vi "RPC_Demo.vi"(11 "Sender":string="RPC Demo") -> ()   [LabVIEW 2014]
uses:
  <vilib>/Utility/miscctls.llb/LVPointTypeDef.ctl
  TSMaster_API/RPC/Typedef/RPC Data.ctl
  <vilib>/Utility/miscctls.llb/LVComboBoxStrsAndValuesArrayTypeDef.ctl
  TSMaster_API/RPC/Typedef/RPC_API_param.ctl
panel:
  out "Connect?":bool
  in  "Disconnect":bool
  in  "TSMaster Proj List":string(combo)
  out "Data out":T1
  in  "选项卡控件":enum32{"Setting", "RPC"}(tab)
  in  "DLL_PATH":path
  in  "API_Call":bool
  in  "API_param":T2
  out "Value":dbl
  in  "Set System Var":bool
  in  "Get System Var":bool
  in  "Var Name":string
  in  "Value_Set":string
  in  "Config":bool
  in  "Connect":bool
  in  "Creat error":bool
  in  "log":i32(listbox)
  in  "Quit":bool
  # "RPC Demo"
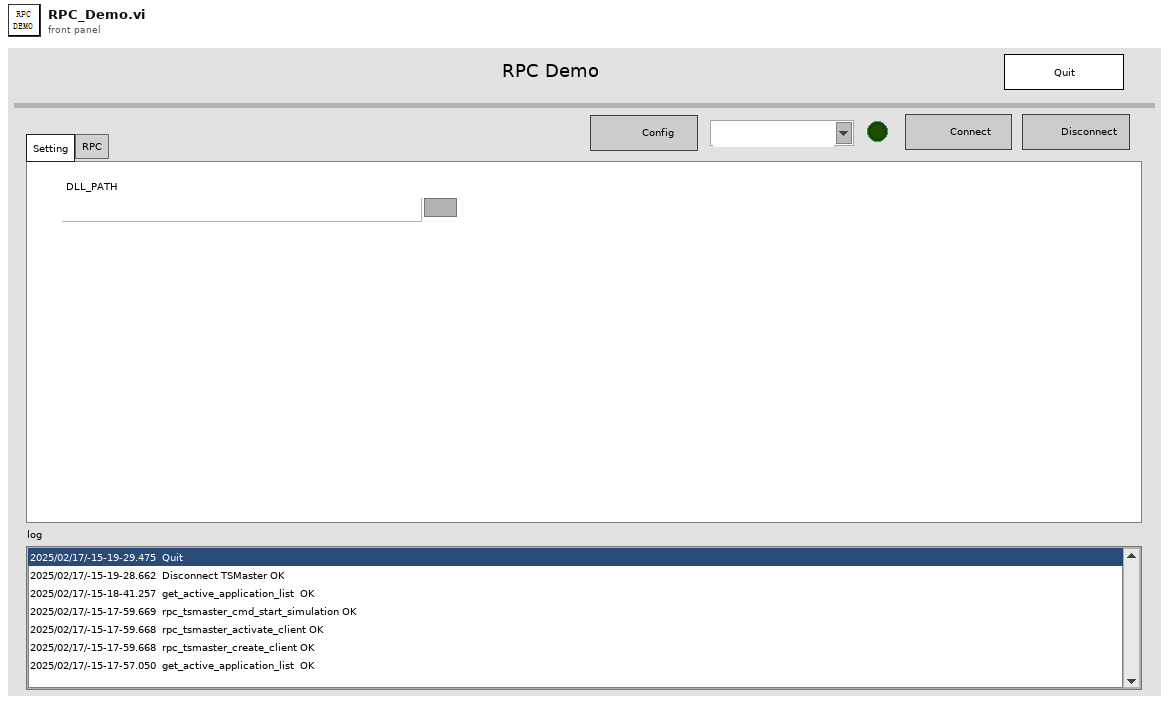
[diagram p1: front panel]
types:
  T1 = typedef "RPC Data.ctl" = cluster{"Communication message":cluster{"Sender":string, "receiver":string, "message":string, "data":variant}, "error in":errorcluster, "Data":cluster{"Config parameter":cluster{"DLL_PATH":path}, "AHandle":i32, "TSMaster Proj":string, "Var Name":string, "API_param":T2}}
  T2 = typedef "RPC_API_param.ctl" = cluster{"AAPIName":string, "AArgCount":i32, "AArgCapacity":i32, "AArgs":string}
  T3 = cluster{"Sender":string, "receiver":string, "message":string, "data":variant}
  T4 = typedef "LVComboBoxStrsAndValuesArrayTypeDef.ctl" = cluster{"String":string, "Value":string}[]
  T5 = typedef "LVPointTypeDef.ctl" = cluster{"Horizontal":i16, "Vertical":i16}
  T6 = cluster{"Config parameter":cluster{"DLL_PATH":path}, "AHandle":i32, "TSMaster Proj":string, "Var Name":string, "API_param":T2}
  T7 = enum32{"invalid app kind", "Development System", "Run Time System", "Student Edition", "Embedded LabVIEW", "Evaluation", "Custom"}
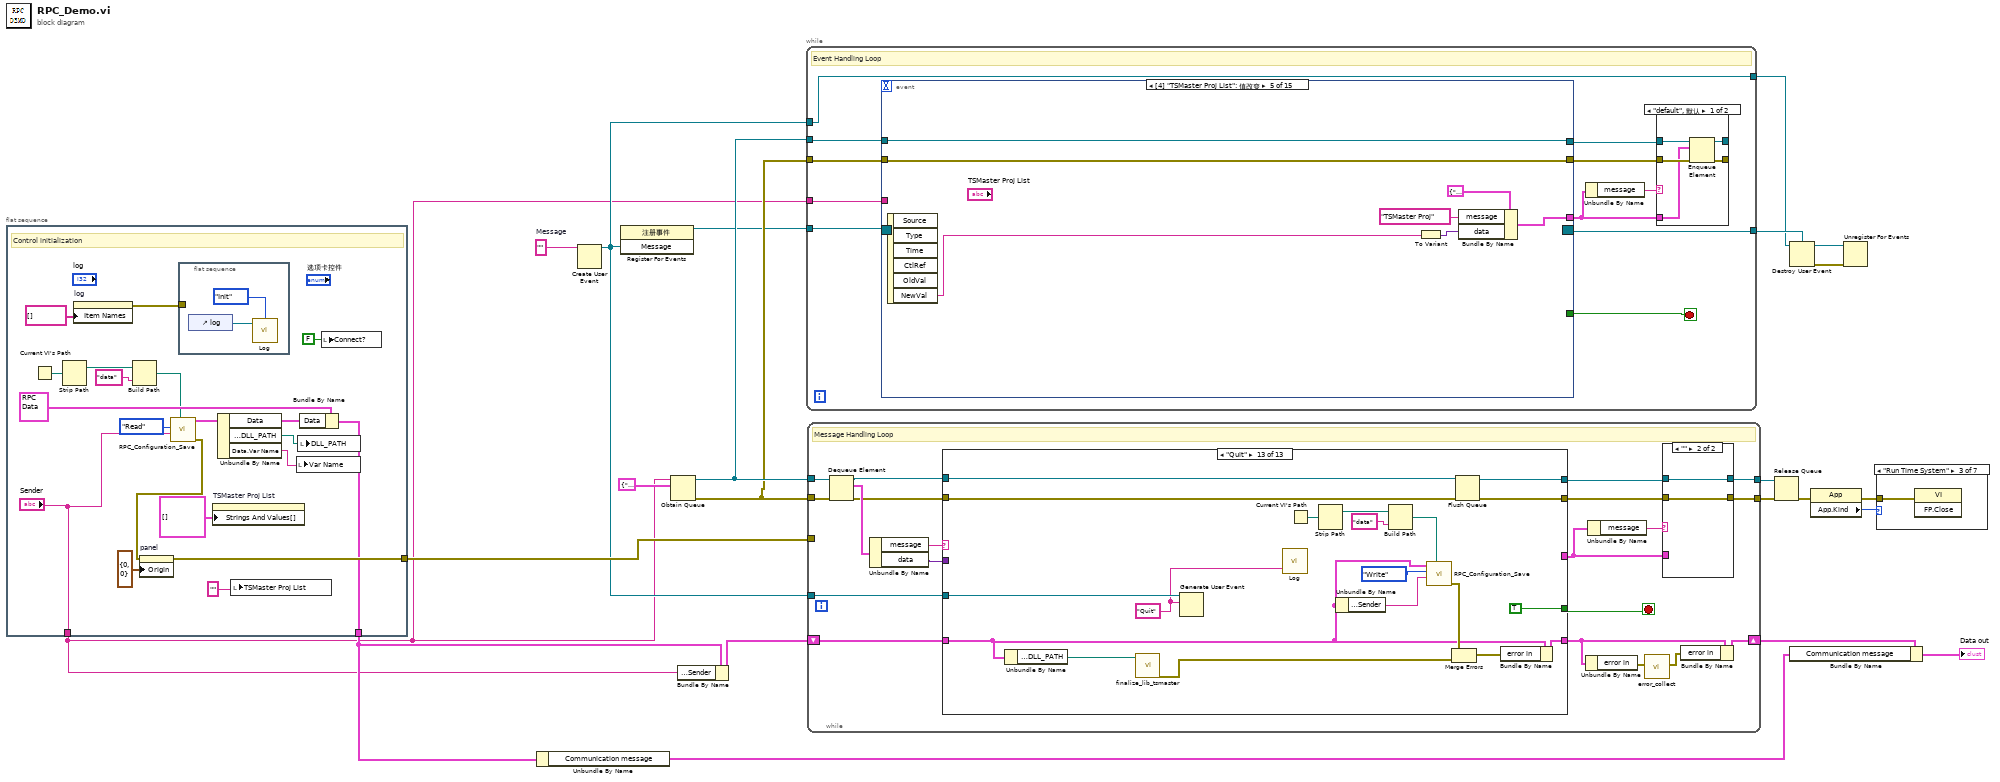
[diagram p0: block diagram]
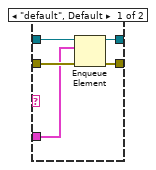
[diagram p8: hidden frame]
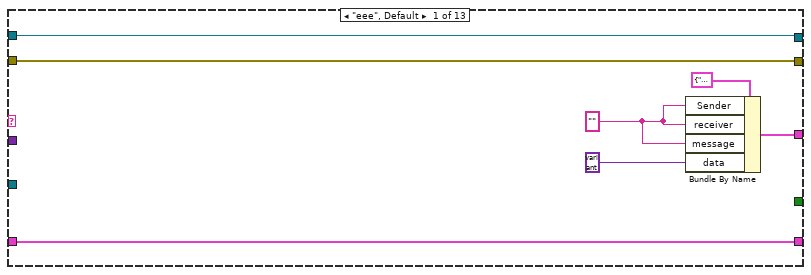
[diagram p9: hidden frame]
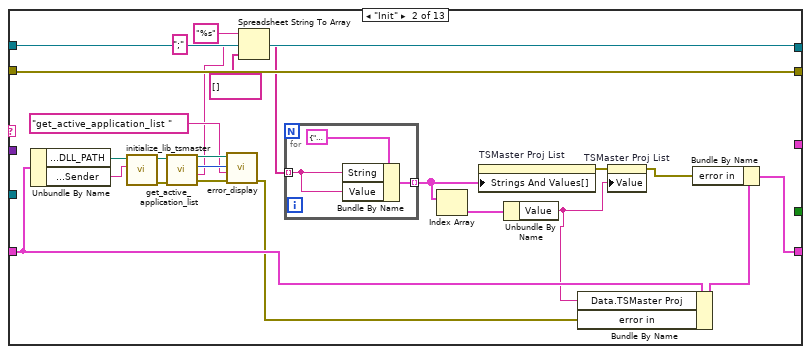
[diagram p10: hidden frame]
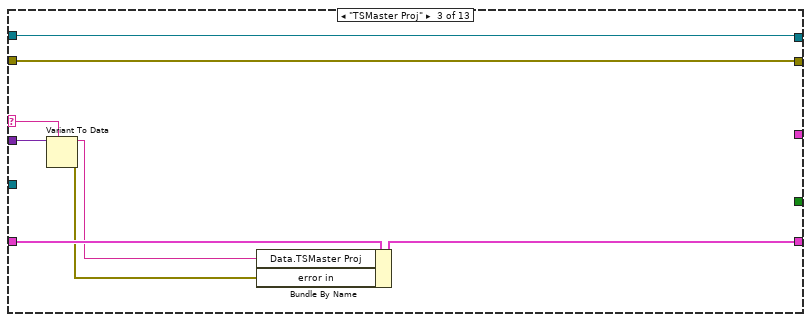
[diagram p11: hidden frame]
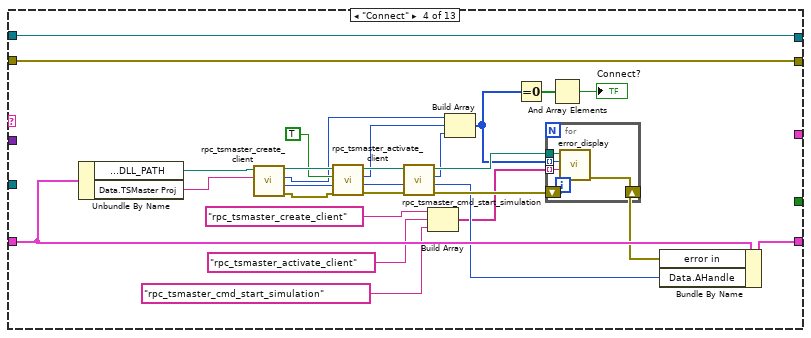
[diagram p12: hidden frame]
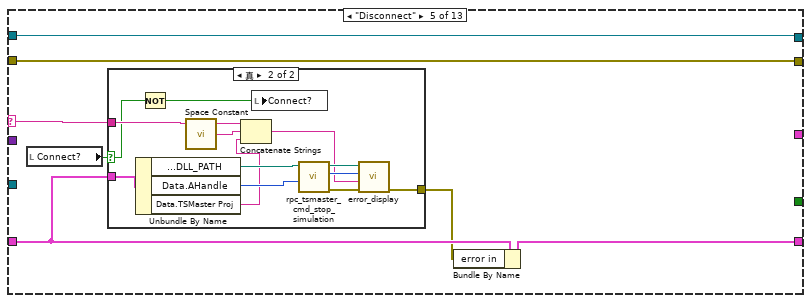
[diagram p13: hidden frame]
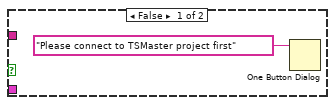
[diagram p14: hidden frame]
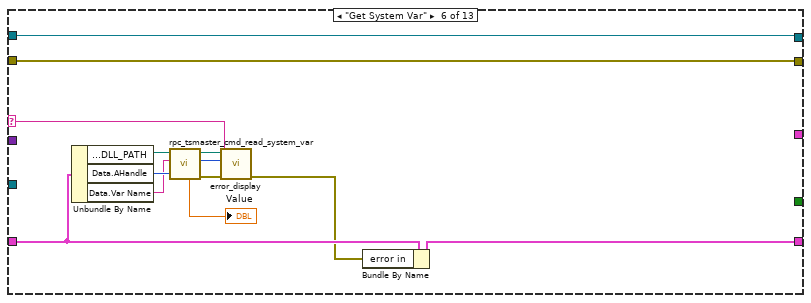
[diagram p15: hidden frame]
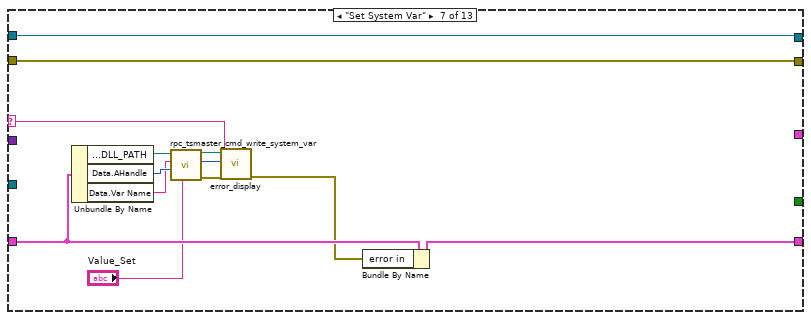
[diagram p16: hidden frame]
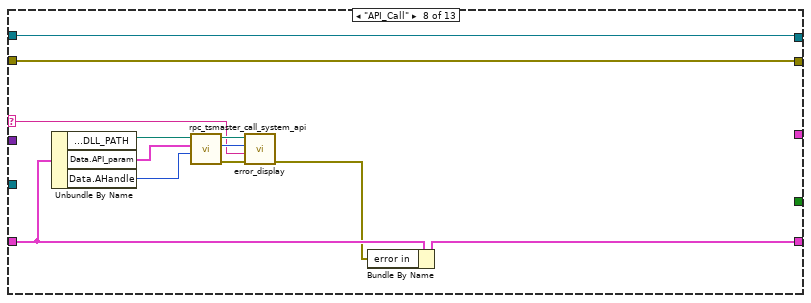
[diagram p17: hidden frame]
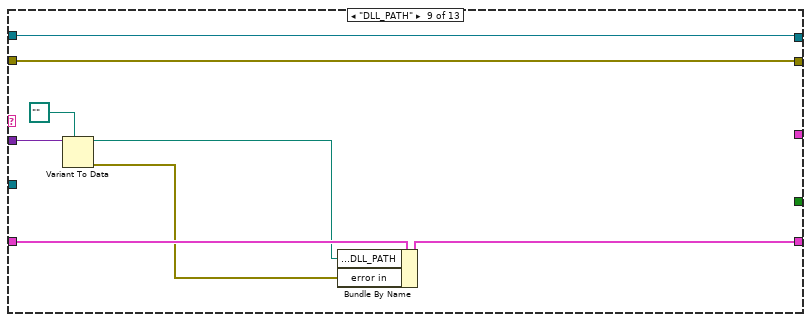
[diagram p18: hidden frame]
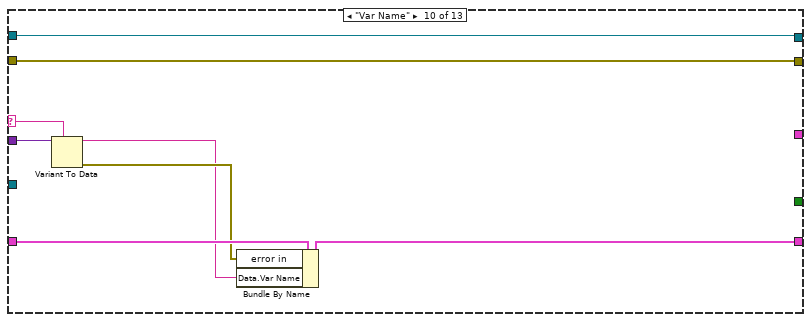
[diagram p19: hidden frame]
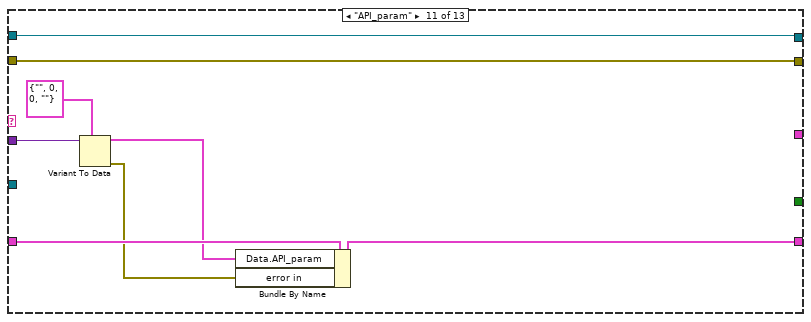
[diagram p20: hidden frame]
diagram:
  w12 = ""  # Message
  n1 = flat-sequence {
    tunnel: [w40] -> w10
    tunnel: [w30] -> w2
    tunnel: ["Sender"] -> w1
    frame #0 {
      # "Control initialization"
      n2 = Current VI's Path() -> (path=w35:path)
      n3 = Strip Path(path=w35) -> (stripped path=w33:path)  [unwired: 1 out]
      n4 = property on="log" class="LstBox (严格)"("Item Names"=string[] [] ("项名")) -> (error out=w38:errorcluster)  [unwired: 2 in, 1 out]
      n5 = Build Path(base path=w33, name or relative path="data") -> (appended path=w32:path)
      n6 = call "RPC_Configuration_Save.vi"("path"=w32, "Config Name"="Sender", "Read/Write"=enum16{"Read", "Write"}."Read") -> ("error in (no error)"=w31:errorcluster, "Data out"=w29:T1)  [unwired: 6 in, 1 out]
      n7 = property on="panel" class="Pane"(error in=w31, "Origin"=T5 {"Horizontal"=0, "Vertical"=0} ("原点")) -> (error out=w40:errorcluster)  [unwired: 1 in, 1 out]
      n8 = flat-sequence {
        tunnel: w38 -> [_]
        frame #0 {
          n9 = control-ref of="log"() -> (w42:refnum<vi>)
          n10 = call "Log.vi"("Method"=enum16{"Init", "Log"}."Init", "ListBox in"=w42) -> ()  [unwired: 2 in]
        }
      }
      n11 = property on="TSMaster Proj List" class="CmbBox"("Strings And Values[]"=T4 [] ("字符串与值[]")) -> ()  [unwired: 2 in, 2 out]
      n12 = Unbundle By Name(w29) -> ("Data"=w28:T6, "Data.Config parameter.DLL_PATH"=w27:path, "Data.Var Name"=w22:string)
      n13 = local write "TSMaster Proj List"("") -> ()
      n14 = local write "Var Name"(w22) -> ()
      n15 = local write "DLL_PATH"(w27) -> ()
      n16 = Bundle By Name(cluster=T1 {"Communication message"={"Sender"="", "receiver"="", "message"="", "data"=variant}, "error in"={"status"=FALSE, "code"=0, "source"=""}, "Data"={"Config parameter"={"DLL_PATH"=path ""}, "AHandle"=0, "TSMaster Proj"="", "Var Name"="", "API_param"={"AAPIName"="", "AArgCount"=0, "AArgCapacity"=0, "AArgs"=""}}} ("Data"), "Data"=w28) -> (w30:T1)
      n17 = local write "Connect?"(FALSE ("Connect?")) -> ()
    }
  }
  n18 = Unbundle By Name(w2) -> ("Communication message"=w4:T3)
  n19 = Create User Event(user event datatype=w12) -> (user event=w7:refnum<user-event>)  [unwired: 1 in, 1 out]
  n20 = register-events(w7) -> (reference out=w11:refnum<event-registration>)  [unwired: 2 in, 1 out]
  n21 = Obtain Queue(name (unnamed)=w1, element data type=T3 {"Sender"="", "receiver"="", "message"="", "data"=variant} ("Communication message")) -> (queue out=w21:refnum<queue>, error out=w14:errorcluster)  [unwired: 3 in, 1 out]
  n22 = Bundle By Name(cluster=w2, "Communication message.Sender"=w1) -> (w13:T1)
  n23 = while {
    tunnel: w21 -> [w53]
    tunnel: w14 -> [w51]
    tunnel: w1 -> [w47]
    tunnel: w11 -> [w46]
    tunnel: [w45] -> w9
    tunnel: w7 -> [w44]
    tunnel: [w44] -> w6
    stop <- w54 stop-if-true
    # "Event Handling Loop"
    n24 = event shown="[4] \"TSMaster Proj List\": 值改变" {
      selector: w46 -> [_ _ _ _ _ _ _ _ _ _ _ _ _ _ _]
      dyn-events: [_ _ _ _ _ _ _ _ _ _ _ _ _ _ _] -> w45
      timeout: _ -> [_ _ _ _ _ _ _ _ _ _ _ _ _ _ _]
      tunnel: [_ _ _ _ _ _ _ _ _ _ _ _ w129 w134 _] -> w54
      tunnel: w53 -> [w64 w71 w78 w83 w90 w95 w100 w105 w110 w115 w122 w127 w132 w137 w144]
      tunnel: [w64 w71 w78 w83 w90 w95 w100 w105 w110 w115 w122 w127 w132 w135 w144] -> w52
      tunnel: [T3 {"Sender"="", "receiver"="", "message"="", "data"=variant} ("Communication message") w67 w73 w79 w86 w91 w96 w101 w106 w111 w118 w125 _ _ w140] -> w49
      tunnel: [w63 w70 w77 w82 w89 w94 w99 w104 w109 w114 w121 w123 w128 w133 w143] -> w50
      tunnel: w51 -> [w63 w70 w77 w82 w89 w94 w99 w104 w109 w114 w121 w123 w128 w133 w143]
      tunnel: w47 -> [_ _ _ _ _ _ _ _ _ _ _ _ _ _ _]
      event Timeout {
        n25 = event-data() -> ()  [unwired: 1 in, 3 out]
      }
      event "DLL_PATH": Value Change {
        n26 = event-data() -> ("NewVal"=w65:path)  [unwired: 1 in, 5 out]
        n27 = To Variant(anything=w65) -> (Variant=w66:variant)
        n28 = Bundle By Name(cluster=T3 {"Sender"="", "receiver"="", "message"="", "data"=variant} ("Communication message"), "message"="DLL_PATH" ("Sender"), "data"=w66) -> (w67:T3)
      }
      event "Var Name": Value Change {
        n29 = event-data() -> ("NewVal"=w72:string)  [unwired: 1 in, 5 out]
        n30 = To Variant(anything=w72) -> (Variant=w74:variant)
        n31 = Bundle By Name(cluster=T3 {"Sender"="", "receiver"="", "message"="", "data"=variant} ("Communication message"), "message"="Var Name" ("Sender"), "data"=w74) -> (w73:T3)
      }
      event "Config": Value Change {
        n32 = event-data() -> ()  [unwired: 1 in, 6 out]
        n33 = Bundle By Name(cluster=T3 {"Sender"="", "receiver"="", "message"="", "data"=variant} ("Communication message"), "message"="Init" ("Sender")) -> (w79:T3)
      }
      event "TSMaster Proj List": Value Change {
        n34 = event-data() -> ("NewVal"=w84:string)  [unwired: 1 in, 5 out]
        n35 = To Variant(anything=w84) -> (Variant=w85:variant)
        n36 = Bundle By Name(cluster=T3 {"Sender"="", "receiver"="", "message"="", "data"=variant} ("Communication message"), "message"="TSMaster Proj" ("Sender"), "data"=w85) -> (w86:T3)
      }
      event "Connect": Value Change {
        n37 = event-data() -> ()  [unwired: 1 in, 6 out]
        n38 = Bundle By Name(cluster=T3 {"Sender"="", "receiver"="", "message"="", "data"=variant} ("Communication message"), "message"="Connect" ("Sender")) -> (w91:T3)
      }
      event "Disconnect": Value Change {
        n39 = event-data() -> ()  [unwired: 1 in, 6 out]
        n40 = Bundle By Name(cluster=T3 {"Sender"="", "receiver"="", "message"="", "data"=variant} ("Communication message"), "message"="Disconnect" ("Sender")) -> (w96:T3)
      }
      event "Get System Var": Value Change {
        n41 = event-data() -> ()  [unwired: 1 in, 1 out]
        n42 = Bundle By Name(cluster=T3 {"Sender"="", "receiver"="", "message"="", "data"=variant} ("Communication message"), "message"="Get System Var" ("Sender")) -> (w101:T3)
      }
      event "Set System Var": Value Change {
        n43 = event-data() -> ()  [unwired: 1 in, 6 out]
        n44 = Bundle By Name(cluster=T3 {"Sender"="", "receiver"="", "message"="", "data"=variant} ("Communication message"), "message"="Set System Var" ("Sender")) -> (w106:T3)
      }
      event "API_Call": Value Change {
        n45 = event-data() -> ()  [unwired: 1 in, 6 out]
        n46 = Bundle By Name(cluster=T3 {"Sender"="", "receiver"="", "message"="", "data"=variant} ("Communication message"), "message"="API_Call" ("Sender")) -> (w111:T3)
      }
      event Value Change {
        n47 = event-data() -> ("NewVal"=w116:T2)  [unwired: 1 in, 5 out]
        n48 = To Variant(anything=w116) -> (Variant=w117:variant)
        n49 = Bundle By Name(cluster=T3 {"Sender"="", "receiver"="", "message"="", "data"=variant} ("Communication message"), "message"="API_param" ("Sender"), "data"=w117) -> (w118:T3)
      }
      event "Quit": Value Change {
        n50 = event-data() -> ()  [unwired: 1 in, 6 out]
        n51 = Bundle By Name(cluster=T3 {"Sender"="", "receiver"="", "message"="", "data"=variant} ("Communication message"), "message"="Quit" ("Sender")) -> (w125:T3)
      }
      event User Event {
        n52 = event-data() -> ("Message"=w131:string)  [unwired: 1 in]
        n53 = Equal?(x=w131, y="Quit") -> (x = y?=w129:bool)
      }
      event Panel Close? {
        w134 = TRUE ("放弃？")
        n54 = event-data() -> ()  [unwired: 1 in, 4 out]
        n55 = Enqueue Element(queue=w137, element=T3 {"Sender"="", "receiver"="", "message"="Quit", "data"=variant} ("Communication message")) -> (queue out=w135:refnum<queue>)  [unwired: 2 in, 2 out]
        n56 = event-data("Discard?"=w134) -> ()  [unwired: 1 in, 1 out]
      }
      event "Creat error": Value Change {
        n57 = event-data() -> ()  [unwired: 1 in, 6 out]
        n58 = To Variant(anything=errorcluster {"status"=TRUE, "code"=709394, "source"="This is a error demo"}) -> (Variant=w138:variant)
        n59 = Bundle By Name(cluster=T3 {"Sender"="", "receiver"="", "message"="", "data"=variant} ("Communication message"), "message"="Creat error" ("Sender"), "data"=w138) -> (w140:T3)
      }
    }
    n60 = Unbundle By Name(w49) -> ("message"=w48:string)
    n61 = case shown="\"default\", 默认" w48 {
      tunnel: w52 -> [w59 w61]
      tunnel: w50 -> [w58 w60]
      tunnel: w49 -> [w57 _]
      tunnel: [w56 w61] -> _
      tunnel: [w55 w60] -> _
      frame "default", Default {
        n62 = Enqueue Element(queue=w59, element=w57, error in (no error)=w58) -> (queue out=w56:refnum<queue>, error out=w55:errorcluster)  [unwired: 1 in, 1 out]
      }
      frame "" {
      }
    }
  }
  n63 = while {
    tunnel: w21 -> [w164]
    tunnel: w14 -> [w163]
    tunnel: [w155] -> w20
    tunnel: [w154] -> w19
    shift-right: [w146] -> w5
    shift-left: w13 -> [w150]
    tunnel: w10 -> [_]
    tunnel: w7 -> [w149]
    stop <- w153 stop-if-true
    # "Message Handling Loop"
    n64 = Dequeue Element(queue=w164, error in (no error)=w163) -> (queue out=w160:refnum<queue>, element=w162:T3, error out=w159:errorcluster)  [unwired: 1 in, 1 out]
    n65 = Unbundle By Name(w162) -> ("message"=w161:string, "data"=w156:variant)
    n66 = case shown="\"Quit\"" w161 {
      selector: w161 -> [_ _ w209 _ w249 w271 w289 w295 _ w316 _ _ _]
      tunnel: [w178 w202 w213 w240 w252 w279 w292 w304 w312 w320 w328 w335 w353] -> w158
      tunnel: w160 -> [w178 w202 w213 w240 w252 w279 w292 w304 w312 w320 w328 w335 w352]
      tunnel: w159 -> [w177 w201 w212 w239 w251 w278 w291 w303 w311 w319 w327 w334 w350]
      tunnel: [w177 w201 w212 w239 w251 w278 w291 w303 w311 w319 w327 w334 w351] -> w157
      tunnel: w156 -> [_ _ w210 _ _ _ _ _ w309 w317 w325 w332 _]
      tunnel: [_ _ _ _ _ _ _ _ _ _ _ _ TRUE] -> w153
      tunnel: [w175 _ _ _ _ _ _ _ _ _ _ _ _] -> w152
      tunnel: [w172 w192 w208 w227 w248 w270 w288 w294 w307 w315 w323 w330 w342] -> w148
      tunnel: w150 -> [w172 w200 w211 w238 w250 w277 w290 w302 w310 w318 w326 w333 w339]
      tunnel: w149 -> [_ _ _ _ _ _ _ _ _ _ _ _ w349]
      frame "eee", Default {
        w173 = ""
        n67 = Bundle By Name(cluster=T3 {"Sender"="", "receiver"="", "message"="", "data"=variant} ("Communication message"), "Sender"=w173, "receiver"=w173, "message"=w173, "data"=variant) -> (w175:T3)
      }
      frame "Init" {
        n68 = Unbundle By Name(w200) -> ("Data.Config parameter.DLL_PATH"=w199:path, "Communication message.Sender"=w198:string)
        n69 = call "initialize_lib_tsmaster.vi"("AppName"=w198, "Path input"=w199) -> ("error output"=w196:errorcluster, "Path output"=w197:path)  [unwired: 8 in]
        n70 = call "get_active_application_list.vi"("error in"=w196, "path in"=w197) -> ("error out"=w194:errorcluster, "ATSMasterAppNames"=w187:string, "return"=w193:i32, "path out"=w195:path)  [unwired: 6 in]
        n71 = call "error_display.vi"("error in"=w194, "Action name"="get_active_application_list ", "return"=w193, "DLL path"=w195) -> ("error out"=w179:errorcluster)  [unwired: 6 in, 1 out]
        n72 = Spreadsheet String To Array(delimiter (Tab)=";" ("分隔符(Tab)"), format string="%s", spreadsheet string=w187, array type (2D Dbl)=string[] []) -> (array=w186:string[])
        n73 = for {
          tunnel: w186 -> [w204] mode=indexing
          tunnel: [w203] -> w184 mode=indexing
          n74 = Bundle By Name(cluster=cluster{"String":string, "Value":string} {"String"="", "Value"=""}, "String"=w204, "Value"=w204) -> (w203:cluster{"String":string, "Value":string})
        }
        n75 = Index Array(array=w184) -> (element=w183:cluster{"String":string, "Value":string})  [unwired: 1 in]
        n76 = property on="TSMaster Proj List" class="CmbBox"("Strings And Values[]"=w184) -> (error out=w185:errorcluster)  [unwired: 2 in, 1 out]
        n77 = Unbundle By Name(w183) -> ("Value"=w180:string)
        n78 = Bundle By Name(cluster=w200, "Data.TSMaster Proj"=w180, "error in"=w179) -> (w181:T1)
        n79 = property on="TSMaster Proj List" class="CmbBox"(error in=w185, "Value"=w180) -> (error out=w182:errorcluster)  [unwired: 1 in, 1 out]
        n80 = Bundle By Name(cluster=w181, "error in"=w182) -> (w192:T1)
      }
      frame "TSMaster Proj" {
        n81 = Variant To Data(type=w209, Variant=w210) -> (data=w207:string, error out=w206:errorcluster)  [unwired: 1 in]
        n82 = Bundle By Name(cluster=w211, "Data.TSMaster Proj"=w207, "error in"=w206) -> (w208:T1)
      }
      frame "Connect" {
        n83 = Unbundle By Name(w238) -> ("Data.Config parameter.DLL_PATH"=w237:path, "Data.TSMaster Proj"=w217:string)
        n84 = call "rpc_tsmaster_create_client.vi"("AppName"=w217, "Path input"=w237) -> ("error output"=w234:errorcluster, "AHandle"=w231:i32, "return"=w224:i32, "Path output"=w236:path)  [unwired: 6 in]
        n85 = call "rpc_tsmaster_activate_client.vi"("error in (no error)"=w234, "AHandle"=w231, "AActivate"=TRUE, "Path input"=w236) -> ("error output"=w233:errorcluster, "AHandle 2"=w229:i32, "return"=w223:i32, "Path output"=w235:path)  [unwired: 4 in]
        n86 = call "rpc_tsmaster_cmd_start_simulation.vi"("error in (no error)"=w233, "AHandle"=w229, "路径输入"=w235) -> ("error out"=w232:errorcluster, "AHandle 2"=w225:u32, "return"=w222:i32, "路径输出"=w228:path)  [unwired: 5 in]
        n87 = Build Array("rpc_tsmaster_create_client", "rpc_tsmaster_activate_client", "rpc_tsmaster_cmd_start_simulation") -> (w218:string[])
        n88 = Build Array(w224, w223, w222) -> (w216:i32[])
        n89 = Equal To 0?(x=w216) -> (x = 0?=w215:bool[])
        n90 = for {
          tunnel: w228 -> [w244]
          shift-right: [w243] -> w226
          shift-left: w232 -> [w245]
          tunnel: w216 -> [w242] mode=indexing
          tunnel: w218 -> [w241] mode=indexing
          n91 = call "error_display.vi"("error in"=w245, "Action name"=w241, "return"=w242, "DLL path"=w244) -> ("error out"=w243:errorcluster)  [unwired: 6 in, 1 out]
        }
        n92 = And Array Elements(Boolean array=w215) -> (logical AND=→"Connect?":bool)
        n93 = Bundle By Name(cluster=w238, "error in"=w226, "Data.AHandle"=w225) -> (w227:T1)
      }
      frame "Disconnect" {
        n94 = local read "Connect?"() -> (w246:bool)
        n95 = case shown="真" w246 {
          selector: w246 -> [_ w255]
          tunnel: w250 -> [_ w266]
          tunnel: w249 -> [_ w260]
          tunnel: [_ w259] -> w247
          frame False {
            n96 = One Button Dialog(message="Please connect to TSMaster project first" ("消息")) -> ()  [unwired: 1 in, 1 out]
          }
          frame True {
            n97 = Unbundle By Name(w266) -> ("Data.Config parameter.DLL_PATH"=w265:path, "Data.AHandle"=w264:i32, "Data.TSMaster Proj"=w257:string)
            n98 = Not(x=w255) -> (.not. x?=w254:bool)
            n99 = call <vilib>:"Space Constant.vi"() -> ("String"=w256:string)
            n100 = Concatenate Strings(w260, w256, w257) -> (w258:string)
            n101 = local write "Connect?"(w254) -> ()
            n102 = call "rpc_tsmaster_cmd_stop_simulation.vi"("AHandle"=w264, "路径输入"=w265) -> ("error out"=w262:errorcluster, "function return"=w261:i32, "路径输出"=w263:path)  [unwired: 7 in]
            n103 = call "error_display.vi"("error in"=w262, "Action name"=w258, "return"=w261, "DLL path"=w263) -> ("error out"=w259:errorcluster)  [unwired: 6 in, 1 out]
          }
        }
        n104 = Bundle By Name(cluster=w250, "error in"=w247) -> (w248:T1)
      }
      frame "Get System Var" {
        n105 = Unbundle By Name(w277) -> ("Data.Config parameter.DLL_PATH"=w276:path, "Data.AHandle"=w275:i32, "Data.Var Name"=w267:string)
        n106 = call "rpc_tsmaster_cmd_read_system_var.vi"("AHandle"=w275, "ASysVarName"=w267, "Path input"=w276) -> ("error output"=w274:errorcluster, "return"=w272:i32, "Path output"=w273:path, "AValue"=→"Value":dbl)  [unwired: 4 in, 1 out]
        n107 = call "error_display.vi"("error in"=w274, "Action name"=w271, "return"=w272, "DLL path"=w273) -> ("error out"=w269:errorcluster)  [unwired: 6 in, 1 out]
        n108 = Bundle By Name(cluster=w277, "error in"=w269) -> (w270:T1)
      }
      frame "Set System Var" {
        n109 = Unbundle By Name(w290) -> ("Data.Config parameter.DLL_PATH"=w286:path, "Data.AHandle"=w281:i32, "Data.Var Name"=w280:string)
        n110 = call "rpc_tsmaster_cmd_write_system_var.vi"("AValue"="Value_Set", "AHandle"=w281, "ACompleteName"=w280, "Path input"=w286) -> ("error output"=w284:errorcluster, "return"=w283:i32, "Path output"=w285:path)  [unwired: 4 in, 1 out]
        n111 = call "error_display.vi"("error in"=w284, "Action name"=w289, "return"=w283, "DLL path"=w285) -> ("error out"=w287:errorcluster)  [unwired: 6 in, 1 out]
        n112 = Bundle By Name(cluster=w290, "error in"=w287) -> (w288:T1)
      }
      frame "API_Call" {
        n113 = Unbundle By Name(w302) -> ("Data.Config parameter.DLL_PATH"=w301:path, "Data.API_param"=w300:T2, "Data.AHandle"=w299:i32)
        n114 = call "rpc_tsmaster_call_system_api.vi"("AHandle"=w299, "API_param"=w300, "路径输入"=w301) -> ("error out"=w296:errorcluster, "function return"=w297:i32, "路径输出"=w298:path)  [unwired: 6 in]
        n115 = call "error_display.vi"("error in"=w296, "Action name"=w295, "return"=w297, "DLL path"=w298) -> ("error out"=w293:errorcluster)  [unwired: 6 in, 1 out]
        n116 = Bundle By Name(cluster=w302, "error in"=w293) -> (w294:T1)
      }
      frame "DLL_PATH" {
        n117 = Variant To Data(type=path "" ("DLL_PATH"), Variant=w309) -> (data=w306:path, error out=w305:errorcluster)  [unwired: 1 in]
        n118 = Bundle By Name(cluster=w310, "Data.Config parameter.DLL_PATH"=w306, "error in"=w305) -> (w307:T1)
      }
      frame "Var Name" {
        n119 = Variant To Data(type=w316, Variant=w317) -> (data=w313:string, error out=w314:errorcluster)  [unwired: 1 in]
        n120 = Bundle By Name(cluster=w318, "error in"=w314, "Data.Var Name"=w313) -> (w315:T1)
      }
      frame "API_param" {
        n121 = Variant To Data(type=T2 {"AAPIName"="", "AArgCount"=0, "AArgCapacity"=0, "AArgs"=""} ("API_param"), Variant=w325) -> (data=w322:T2, error out=w321:errorcluster)  [unwired: 1 in]
        n122 = Bundle By Name(cluster=w326, "Data.API_param"=w322, "error in"=w321) -> (w323:T1)
      }
      frame "Creat error" {
        n123 = Variant To Data(type=errorcluster {"status"=FALSE, "code"=0, "source"=""} ("error out"), Variant=w332) -> (data=w329:errorcluster)  [unwired: 1 in, 1 out]
        n124 = Bundle By Name(cluster=w333, "error in"=w329) -> (w330:T1)
      }
      frame "Quit" {
        w348 = "Quit" ("y")
        n125 = Unbundle By Name(w339) -> ("Data.Config parameter.DLL_PATH"=w338:path)
        n126 = call "finalize_lib_tsmaster.vi"("Path"=w338) -> ("error out"=w336:errorcluster)  [unwired: 9 in, 1 out]
        n127 = Generate User Event(user event=w349, event data cluster=w348) -> ()  [unwired: 2 in, 2 out]
        n128 = call "Log.vi"("Data"=w348) -> ()  [unwired: 3 in]
        n129 = Current VI's Path() -> (path=w344:path)
        n130 = Strip Path(path=w344) -> (stripped path=w346:path)  [unwired: 1 out]
        n131 = Unbundle By Name(w339) -> ("Communication message.Sender"=w340:string)
        n132 = Build Path(base path=w346, name or relative path="data") -> (appended path=w347:path)
        n133 = call "RPC_Configuration_Save.vi"("path"=w347, "Config Name"=w340, "Read/Write"=enum16{"Read", "Write"}."Write", "Data in"=w339) -> ("error in (no error)"=w341:errorcluster)  [unwired: 5 in, 2 out]
        n134 = Merge Errors(w341, w336) -> (w337:errorcluster)
        n135 = Flush Queue(queue=w352, error in (no error)=w350) -> (queue out=w353:refnum<queue>, error out=w351:errorcluster)  [unwired: 1 out]
        n136 = Bundle By Name(cluster=w339, "error in"=w337) -> (w342:T1)
      }
    }
    n137 = Unbundle By Name(w148) -> ("error in"=w147:errorcluster)
    n138 = Unbundle By Name(w152) -> ("message"=w151:string)
    n139 = call "error_collect.vi"("error in (no error)"=w147) -> ("error IO"=w145:errorcluster)  [unwired: 10 in]
    n140 = case shown="\"\"" w151 {
      tunnel: w158 -> [w169 w171]
      tunnel: w157 -> [w168 w170]
      tunnel: w152 -> [w167 _]
      tunnel: [w166 w171] -> w155
      tunnel: [w165 w170] -> w154
      frame "default", Default {
        n141 = Enqueue Element(queue=w169, element=w167, error in (no error)=w168) -> (queue out=w166:refnum<queue>, error out=w165:errorcluster)  [unwired: 1 in, 1 out]
      }
      frame "" {
      }
    }
    n142 = Bundle By Name(cluster=w148, "error in"=w145) -> (w146:T1)
  }
  n143 = Release Queue(queue=w20, error in (no error)=w19) -> (error out=w18:errorcluster)  [unwired: 1 in, 2 out]
  n144 = Destroy User Event(user event=w6) -> (error out=w8:errorcluster)  [unwired: 1 in]
  n145 = Bundle By Name(cluster=w5, "Communication message"=w4) -> (→"Data out":T1)
  n146 = property class="App"(error in=w18) -> (error out=w17:errorcluster, "App.Kind"=w16:T7)  [unwired: 1 in, 1 out]
  n147 = Unregister For Events(event registration refnum=w9, error in=w8) -> ()  [unwired: 1 out]
  n148 = case shown="\"Run Time System\"" w16 {
    tunnel: w17 -> [_ _ w355 _ _ _ _]
    frame "invalid app kind", Default {
    }
    frame "Development System" {
    }
    frame "Run Time System" {
      n149 = invoke class="VI" method="FP.Close"(error in=w355) -> ()  [unwired: 2 in, 3 out]
    }
    frame "Student Edition" {
    }
    frame "Embedded LabVIEW" {
    }
    frame "Evaluation" {
    }
    frame "Custom" {
    }
  }
